vi "Gen - Get Application Kind.vi"(8 "Error In":errorcluster) -> (0 "Error Out":errorcluster, 3 "Application:Kind":T1(ring))   [LabVIEW 2020]
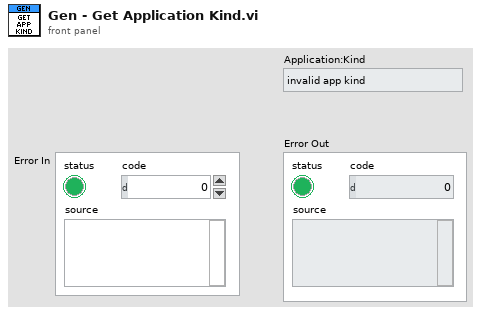
[diagram p1: front panel]
types:
  T1 = enum32{"invalid app kind", "Development System", "Run Time System", "Student Edition", "Embedded LabVIEW", "Evaluation", "Custom"}
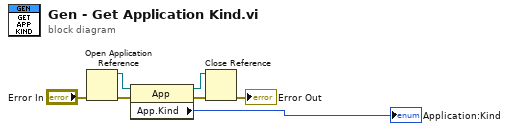
[diagram p0: block diagram]
diagram:
  n1 = Open Application Reference(8:"Error In") -> (0:w6:errorcluster, 3:w2:refnum<vi>)  [unwired: 3 in]
  n2 = property class="App"(reference=w2, error in=w6) -> (reference out=w3:refnum<vi>, error out=w7:errorcluster, "App.Kind"=→"Application:Kind":T1)
  n3 = Close Reference(reference=w3, error in (no error)=w7) -> (error out=→"Error Out":errorcluster)
